vi "ObtainEventLoggerQueue.vi"(8 "Error In":errorcluster) -> (0 "Error Out":errorcluster, 3 "EventLoggerQueue":refnum<queue>)   [LabVIEW 2019, in "EventLogger.lvlib"]
uses:
  EventLogger.lvlib
  Cluster - MessageCluster.ctl
  Enum - Message.ctl
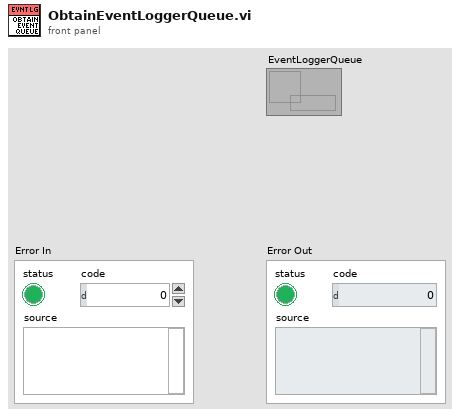
[diagram p1: front panel]
types:
  T1 = typedef "EventLogger.lvlib/Cluster - MessageCluster.ctl" = cluster{"Message":T2, "Data":variant}
  T2 = typedef "EventLogger.lvlib/Enum - Message.ctl" = enum16{"Initialize", "Idle", "CreateLog", "LogStrEvent", "LogErrorEvent", "LogVICall", "Error", "Exit"}
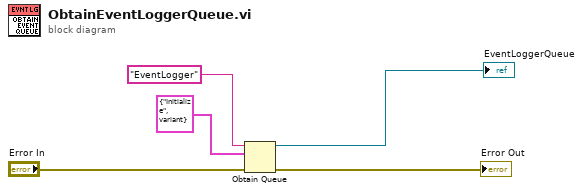
[diagram p0: block diagram]
diagram:
  n1 = Obtain Queue(name (unnamed)="EventLogger", element data type=T1 {"Message"=enum."Initialize", "Data"=variant}, error in (no error)="Error In") -> (queue out=→"EventLoggerQueue":refnum<queue>, error out=→"Error Out":errorcluster)  [unwired: 2 in, 1 out]
